vi "writeToXML.vi"(8 "error in (no error)":errorcluster, 10 "classLabel":string, 11 "PointAdd in":refnum<class "PointAdd.lvclass">) -> (0 "error out":errorcluster, 2 "XML out":string, 3 "PointAdd out":refnum<class "PointAdd.lvclass">)   [LabVIEW 2022 SP3, in "TCSDataDefinitions.lvlib" / "TCSCommand.lvlib" / "PointingFileCommands.lvlib" / "PointAdd.lvclass"]
uses:
  PointAdd.lvclass
  PointingFileCommands/PointingFileCommands.lvclass
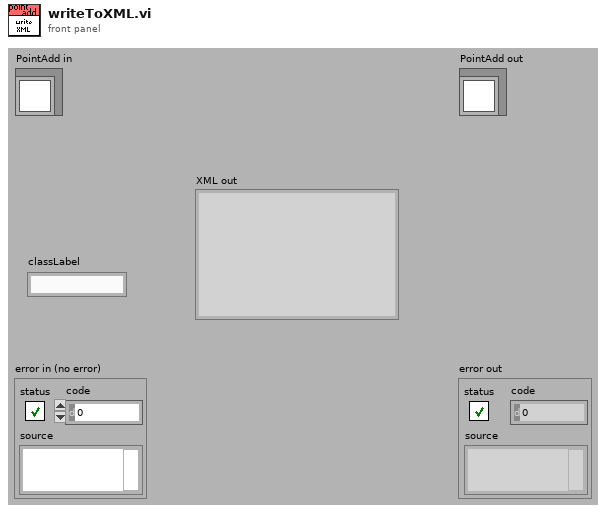
[diagram p1: front panel]
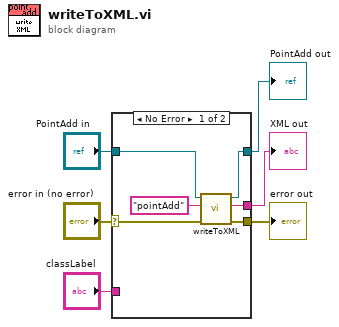
[diagram p0: block diagram]
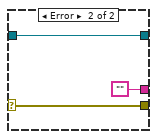
[diagram p2: hidden frame]
diagram:
  n1 = case shown="No Error" "error in (no error)" {
    selector: "error in (no error)" -> [w9 w15]
    tunnel: [w8 w15] -> w5
    tunnel: [w11 w14] -> w3
    tunnel: "PointAdd in" -> [w12 w14]
    tunnel: "classLabel" -> [_ _]
    tunnel: [w10 ""] -> w1
    frame No Error {
      n2 = call-parent "writeToXML.vi"("error in (no error)"=w9, "ClassLabel"="pointAdd", "PointingFileCommands in"=w12) -> ("error out"=w8:errorcluster, "XML out"=w10:string, "PointingFileCommands out"=w11:refnum<class "PointAdd.lvclass">)  [unwired: 6 in]
    }
    frame Error {
    }
  }
  "error out" <- w5
  "PointAdd out" <- w3
  "XML out" <- w1
